vi "matrix_matrix_multiply_SGL.vi"(1 "p":i32, 3 "n":i32, 4 "m":i32, 5 "B":sgl[](array[numeric]), 6 "A":sgl[](array[numeric])) -> (0 "C":sgl[](array[numeric]))   [LabVIEW 2020]
panel:
  in  "accum":sgl format="%#_13g"
  in  "C_type":sgl format="%#_13g"
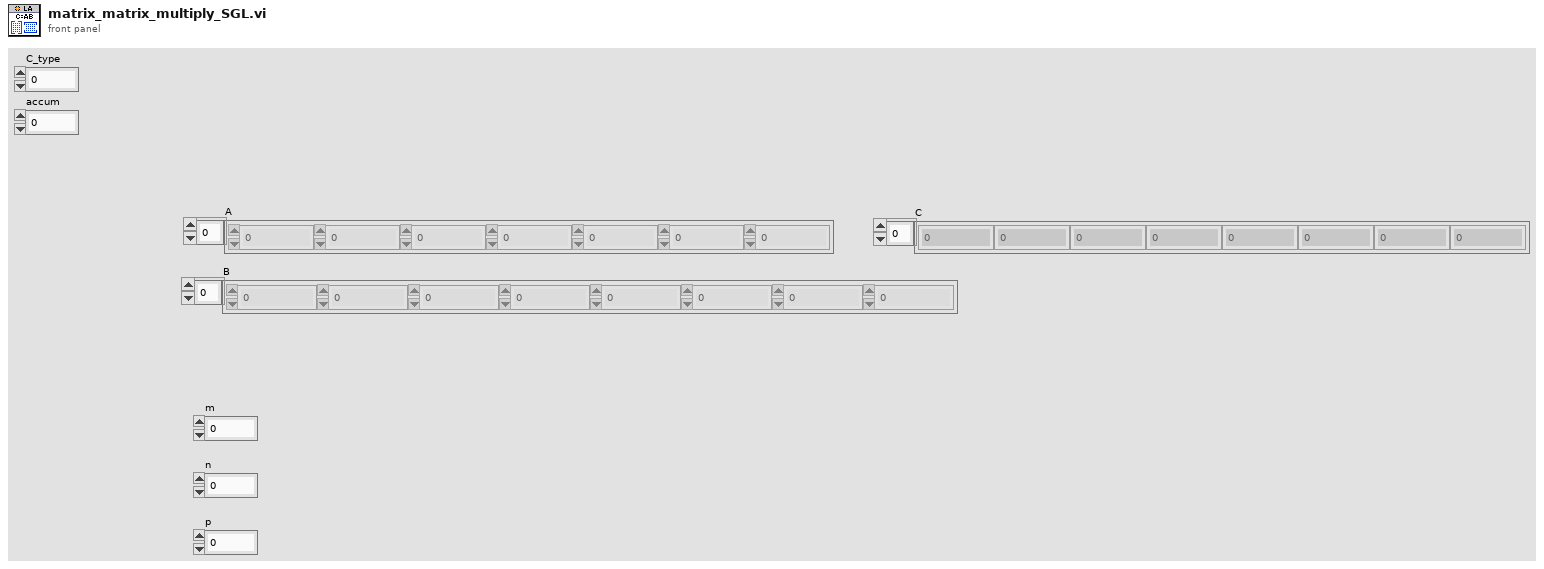
[diagram p1: front panel]
types:
  T1 = enum32{"Extended Precision", "Double Precision", "Single Precision", "Long", "Word", "Byte", "Unsigned Long", "Unsigned Word", "Unsigned Byte", "Complex Extended", "Complex Double", "Complex Single", "Quad", "Unsigned Quad", "Fixed-Point"}
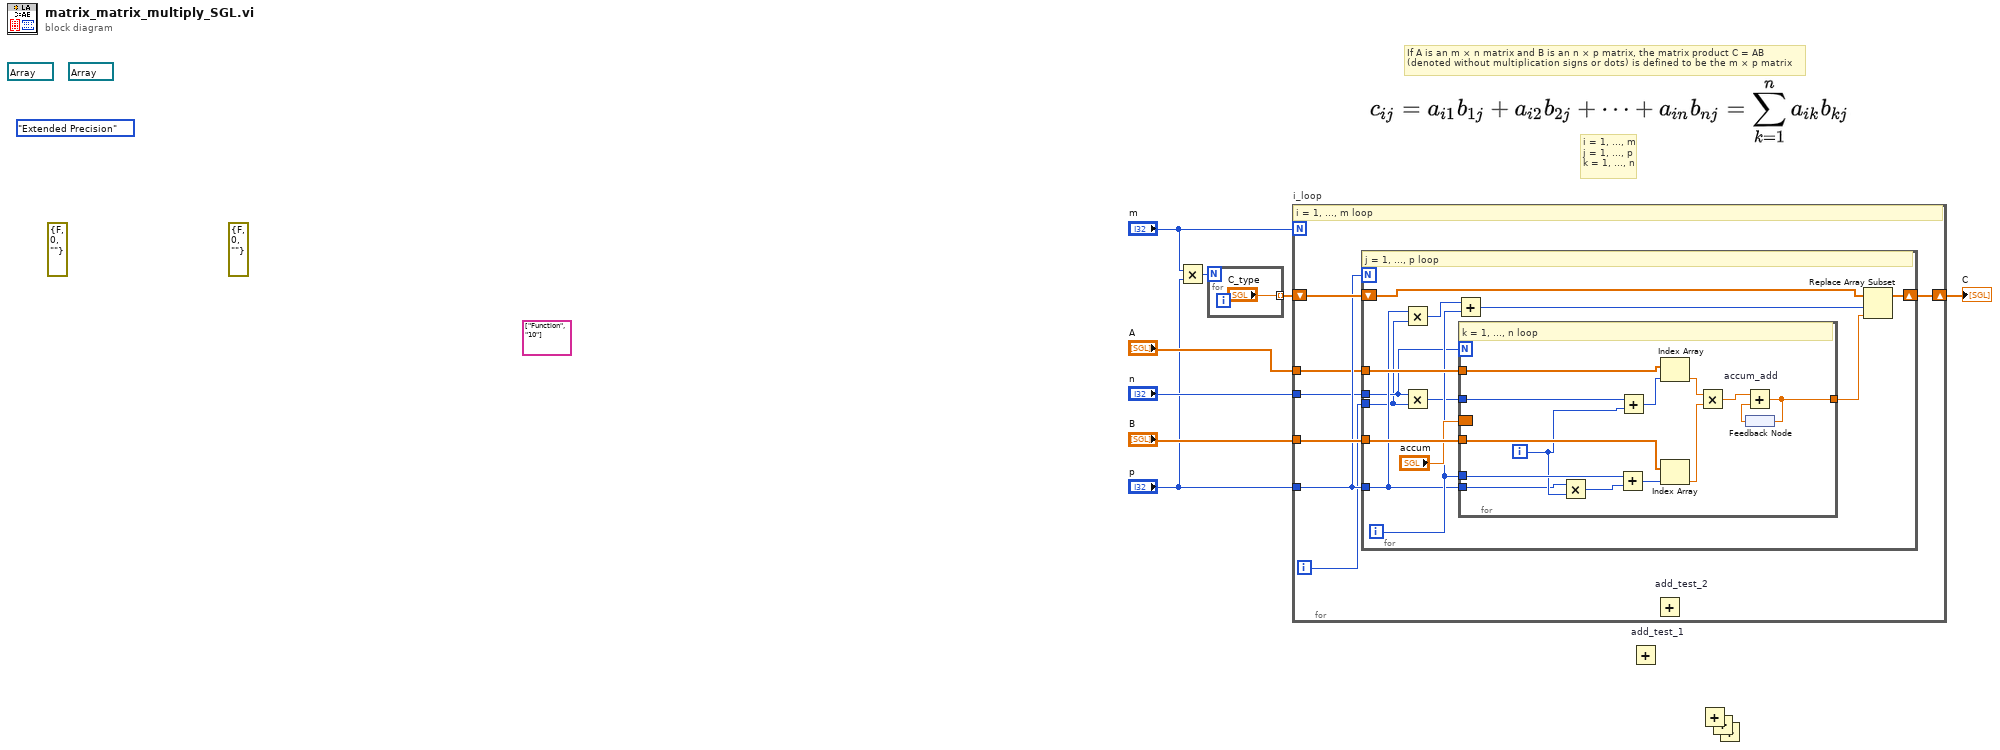
[diagram p0: block diagram]
diagram:
  (unwired) string[][] [["Function", "10"]] ("Traverse All")
  (unwired) refnum<vi> refnum ("Array Ref.")
  (unwired) T1."Extended Precision" ("Representation")
  (unwired) errorcluster {"status"=FALSE, "code"=0, "source"=""} ("error in (no error)")
  (unwired) refnum<vi> refnum ("Ref. Out")
  (unwired) errorcluster {"status"=FALSE, "code"=0, "source"=""} ("error out")
  # "If A is an m × n matrix and B is an n × p matrix, the matrix product C = AB \n(denoted without multiplication signs or dots) is defined to be the m × p matrix"
  # "i = 1, ..., m\nj = 1, ..., p\nk = 1, ..., n"
  n1 = Multiply(x="m", y="p") -> (x*y=w4:i32)
  n2 = for {
    N: w4 -> [_]
    tunnel: ["C_type"] -> w1 mode=indexing
  }
  n3 = for "i_loop" {
    N: "m" -> [_]
    tunnel: "B" -> [w16]
    tunnel: "p" -> [w13]
    tunnel: "A" -> [w12]
    tunnel: "n" -> [w11]
    shift-right: [w14] -> w6
    shift-left: w1 -> [w15]
    i -> [w10]
    # "i = 1, ..., m loop"
    n4 = for {
      N: w13 -> [_]
      tunnel: w12 -> [w29]
      tunnel: w16 -> [w28]
      tunnel: w13 -> [w19]
      shift-right: [w25] -> w14
      shift-left: w15 -> [w26]
      tunnel: w11 -> [w18]
      tunnel: w10 -> [w17]
      i -> [w22]
      # "j = 1, ..., p loop"
      n5 = Multiply(x=w19, y=w17) -> (x*y=w21:i32)
      n6 = Multiply(x=w18, y=w17) -> (x*y=w20:i32)
      n7 = Add(x=w21, y=w22) -> (x+y=w23:i32)
      n8 = for {
        N: w18 -> [_]
        tunnel: w29 -> [w43]
        tunnel: w20 -> [w30]
        tunnel: w28 -> [w42]
        tunnel: w22 -> [w36]
        tunnel: [w37] -> w24
        tunnel: w19 -> [w34]
        border: "accum" -> [_]
        i -> [w35]
        # "k = 1, ..., n loop"
        n9 = Multiply(x=w34, y=w35) -> (x*y=w33:i32)
        n10 = Add(x=w36, y=w33) -> (x+y=w32:i32)
        n11 = Add(x=w30, y=w35) -> (x+y=w31:i32)
        n12 = Index Array(array=w43, index=w31) -> (element=w41:sgl)
        n13 = Index Array(array=w42, index=w32) -> (element=w40:sgl)
        n14 = Multiply(x=w41, y=w40) -> (x*y=w39:sgl)
        n15 = feedback #1() -> (w38:sgl)
        n16 = Add "accum_add"(x=w39, y=w38) -> (x+y=w37:sgl)
        n17 = feedback-in #1(w37) -> ()
      }
      n18 = Replace Array Subset(array=w26, new element=w24, index=w23) -> (w25:sgl[])
    }
    n19 = Add "add_test_2"() -> ()  [unwired: 2 in, 1 out]
  }
  "C" <- w6
  n20 = Add "add_test_1"() -> ()  [unwired: 2 in, 1 out]
  n21 = Add() -> ()  [unwired: 2 in, 1 out]
  n22 = Add() -> ()  [unwired: 2 in, 1 out]
  n23 = Add() -> ()  [unwired: 2 in, 1 out]
